vi "REV ft per s to RPM.vi"() -> ()   [LabVIEW 2020]
panel:
  in  "ft/s":dbl
  out "RPM":dbl
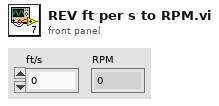
[diagram p1: front panel]
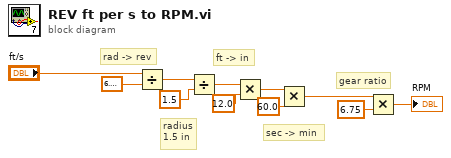
[diagram p0: block diagram]
diagram:
  # "gear ratio"
  # "sec -> min"
  # "ft -> in"
  # "radius\n1.5 in"
  # "rad -> rev"
  n1 = Divide(x="ft/s", y=6.283185307179586) -> (x/y=w10:dbl)
  n2 = Divide(x=w10, y=1.5) -> (x/y=w8:dbl)
  n3 = Multiply(x=w8, y=12.0) -> (x*y=w6:dbl)
  n4 = Multiply(x=w6, y=60.0) -> (x*y=w4:dbl)
  n5 = Multiply(x=w4, y=6.75) -> (x*y=→"RPM":dbl)
